vi "reading spreadsheet.vi"() -> ()   [LabVIEW 2018]
uses:
  <vilib>/Utility/file.llb/Read Delimited Spreadsheet (DBL).vi
panel:
  out "subarray":dbl[](array[numeric])
  out "all rows":dbl[][](array[numeric])
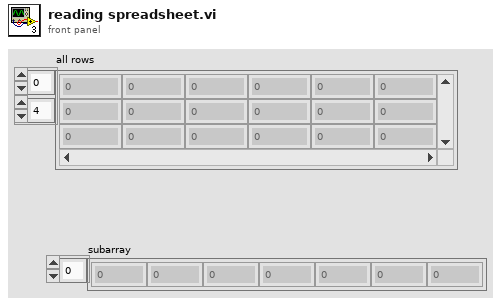
[diagram p1: front panel]
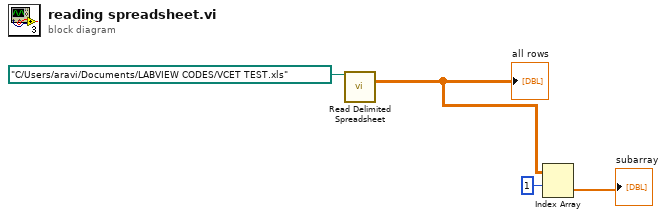
[diagram p0: block diagram]
diagram:
  n1 = call-poly <vilib>:"Read Delimited Spreadsheet.vi"("file path (dialog if empty)"=path "C:/Users/aravi/Documents/LABVIEW CODES/VCET TEST.xls") -> ("all rows"=w3:dbl[][])  [unwired: 9 in, 5 out]
  "all rows" <- w3
  n2 = Index Array "Index Array"(array=w3, index (row)=1) -> (element=→"subarray":dbl[])  [unwired: 1 in]
